vi "RSZVB Get Connector.vi"(8 "error in (no error)":errorcluster {"code" format="%.0x"}, 9 "Port (1)":i32=1, 10 "Channel (1)":i32=1, 11 "VISA session":refnum<visa-resource-name>) -> (0 "error out":errorcluster {"code" format="%.0x"}, 2 "Connector":i32, 3 "dup VISA session":refnum<visa-resource-name>)   [LabVIEW 2011]
doc: "This VI queries a connector type at a specified port <Port> and its gender.\n\nRemote-control command(s):\n[SENSe<Ch>:]CORRection:COLLect:CONNection<port_no>?"
uses:
  _utility/RSZVB Global Data.vi
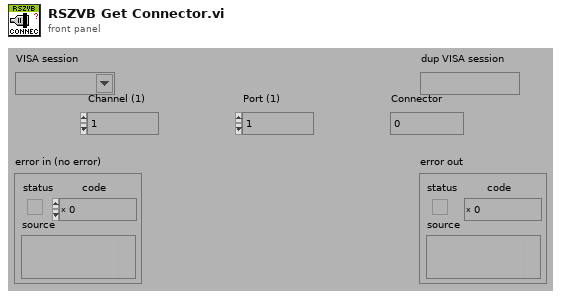
[diagram p1: front panel]
types:
  T1 = cluster{"Error Checking (T: On)":bool, "Installed Options":string[], "Data Valid?":bool, "Ports":i32, "Model":string[], "Option Checking (T: On)":bool}[]
  T2 = cluster{"Error Checking (T: On)":bool, "Installed Options":string[], "Data Valid?":bool, "Ports":i32, "Model":string[], "Option Checking (T: On)":bool}
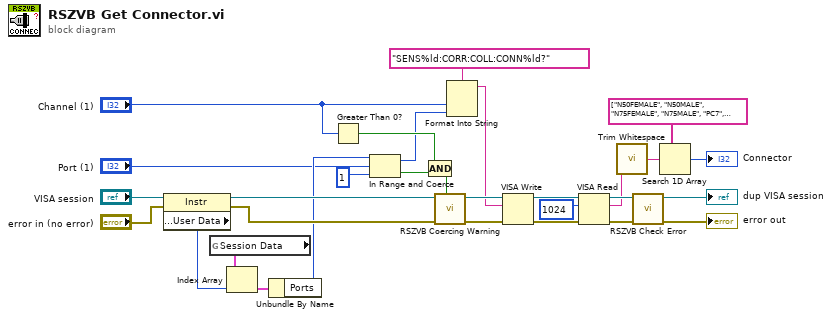
[diagram p0: block diagram]
diagram:
  n1 = property class="Instr"(reference="VISA session", error in="error in (no error)") -> (reference out=w18:refnum<visa-resource-name>, error out=w19:errorcluster, "General Settings:User Data"=w20:u32)
  n2 = global read "RSZVB Global Data.vi" "Session Data"() -> (w21:T1)
  n3 = Index Array(array=w21, index=w20) -> (element=w22:T2)
  n4 = Unbundle By Name(w22) -> ("Ports"=w17:i32)
  n5 = Greater Than 0?(x="Channel (1)") -> (x > 0?=w23:bool)
  n6 = In Range and Coerce(upper limit=w17, x="Port (1)", lower limit=1) -> (coerced(x)=w16:i32, In Range?=w26:bool)
  n7 = Compound Arithmetic op=AND(w23, w26) -> (w25:bool)
  n8 = call "RSZVB Coercing Warning.vi"("In Range?"=w25, "error in (no error)"=w19, "VISA session"=w18) -> ("error out"=w27:errorcluster, "dup VISA session"=w28:refnum<visa-resource-name>)  [unwired: 7 in]
  n9 = Format Into String(format string="SENS%ld:CORR:COLL:CONN%ld?", "Channel (1)", w16) -> (resulting string=w24:string)  [unwired: 2 in, 1 out]
  n10 = VISA Write(VISA resource name=w28, write buffer=w24, error in (no error)=w27) -> (VISA resource name out=w7:refnum<visa-resource-name>, error out=w8:errorcluster)  [unwired: 1 out]
  n11 = VISA Read(VISA resource name=w7, byte count=u32 1024 ("byte count (0)"), error in (no error)=w8) -> (VISA resource name out=w10:refnum<visa-resource-name>, read buffer=w2:string, error out=w9:errorcluster)  [unwired: 1 out]
  n12 = call <vilib>:"Trim Whitespace.vi"("string"=w2) -> ("trimmed string"=w1:string)  [unwired: 1 in]
  n13 = call "RSZVB Check Error.vi"("error in (no error)"=w9, "VISA session"=w10) -> ("error out"=→"error out":errorcluster, "dup VISA session"=→"dup VISA session":refnum<visa-resource-name>)  [unwired: 8 in]
  n14 = Search 1D Array(1D array=string[] ["N50FEMALE", "N50MALE", "N75FEMALE", "N75MALE", "PC7", "PC35FEMALE", "PC35MALE", "PC292FEMALE", "PC292MALE", "UFEMALE1", "UMALE1", "UFEMALE2", "UMALE2", "SMAFEMALE", "SMAMALE", "PC1FEMALE", "PC1MALE", "PC185FEMALE", "PC185MALE", "PC24FEMALE", "PC24MALE"] ("array 2"), element=w1) -> (index of element=→"Connector":i32)  [unwired: 1 in]
